vi "PBcard_select_close.vi"(0 "error in (no error)":errorcluster, 1 "Select Board Indicator":i32) -> (2 "error out":errorcluster)   [LabVIEW 2013]
doc: "This vi sends a software trigger to the PulseBlaster.\n\nIn order to start the PulseBlaster, the following sequence must occur, even if the PulseBlaster is not reprogrammed, but merely retriggered:\n1) Reset the PulseBlaster\n2) Load number of bytes per word\n3) Select Memory device (external or internal)\n4) Clear address counter\n5) Send program finished\n6) Send the \"start\" trigger.\n\nThe inputs should rarely be changed, as they are hardware specific."
uses:
  DeviceVIs/Utils_devs/SpinAPI/SpinAPI-20140801.lvlib
panel:
  out "path out":path
  in  "path in":path=path "C:/SpinCore/SpinAPI/dll/spinapi.dll"
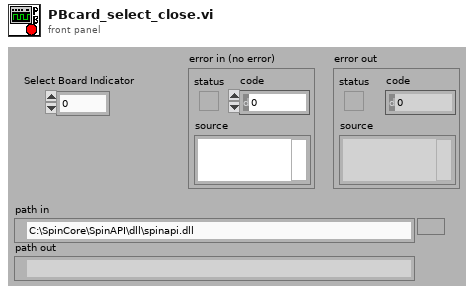
[diagram p1: front panel]
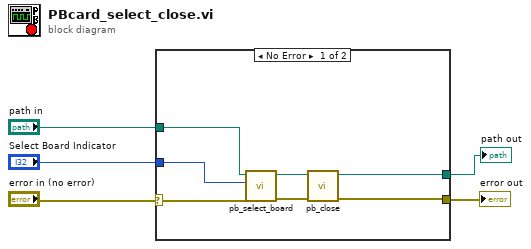
[diagram p0: block diagram]
diagram:
  n1 = case shown="No Error" "error in (no error)" {
    selector: "error in (no error)" -> [w9 w14]
    tunnel: [w8 w14] -> w4
    tunnel: "Select Board Indicator" -> [w10 _]
    tunnel: "path in" -> [w7 w13]
    tunnel: [w6 w13] -> w1
    frame No Error {
      n2 = call "pb_select_board.vi"("error in (no error)"=w9, "board_num"=w10, "path in"=w7) -> ("error out"=w11:errorcluster, "path out"=w12:path)  [unwired: 7 in]
      n3 = call "pb_close.vi"("error in (no error)"=w11, "path in"=w12) -> ("error out"=w8:errorcluster, "path out"=w6:path)  [unwired: 8 in]
    }
    frame Error {
    }
  }
  "error out" <- w4
  "path out" <- w1
